vi "test Get Attribute as JSON Multiple Tables.vi"(11 "Test Case In":refnum<class "Test Config From Excel Table.lvclass">) -> (0 "error out":errorcluster, 3 "Test Case Out":refnum<class "Test Config From Excel Table.lvclass">)   [LabVIEW 2020, in "Test Config From Excel Table.lvclass"]
uses:
  Test Config From Excel Table.lvclass
  C:/Program Files/National Instruments/LabVIEW 2025/vi.lib/Astemes/LUnit/Test Case.lvclass
  Source/Config from Excel Table/Config from Excel Table.lvclass
  <vilib>/Astemes/LUnit/Test Case.lvclass/Test Case.ctl
  <vilib>/JDP Science/JSONtext/JSONtext.lvlib
  <vilib>/Astemes/LUnit/Test Case.lvclass
  <vilib>/Peter/Open Xml/Source/Open Xml.lvlib
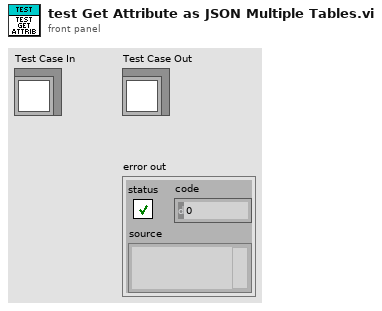
[diagram p1: front panel]
types:
  T1 = cluster{"Sheet Name":string, "Name":string, "Display Name":string, "Range or Cell Address":string}
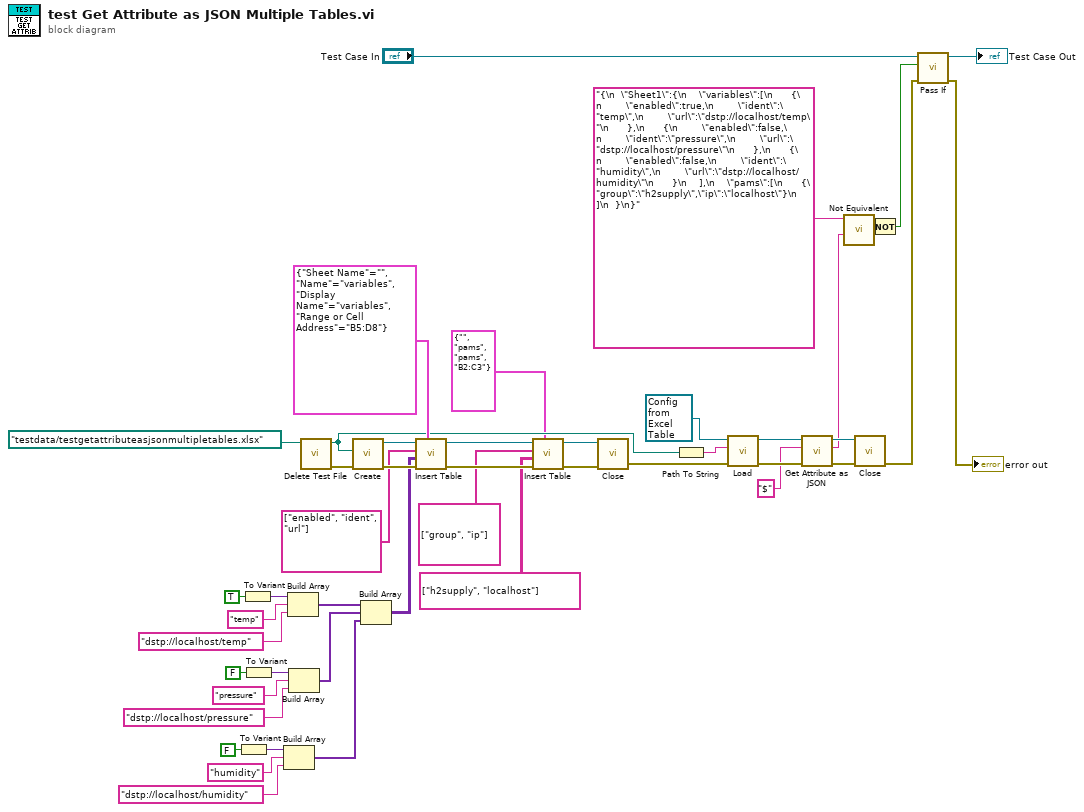
[diagram p0: block diagram]
diagram:
  n1 = To Variant(anything=FALSE) -> (Variant=w20:variant)
  n2 = To Variant(anything=TRUE) -> (Variant=w29:variant)
  n3 = To Variant(anything=FALSE) -> (Variant=w23:variant)
  n4 = Build Array(w20, "humidity", "dstp://localhost/humidity") -> (w16:variant[])
  n5 = Build Array(w29, "temp", "dstp://localhost/temp") -> (w26:variant[])
  n6 = Build Array(w23, "pressure", "dstp://localhost/pressure") -> (w17:variant[])
  n7 = call "Delete Test File.vi"("name or relative path"=path "testdata/testgetattributeasjsonmultipletables.xlsx") -> ("error out"=w34:errorcluster, "deleted path"=w9:path)  [unwired: 9 in]
  n8 = call <vilib>:"Create.vi"("error in"=w34, "Path"=w9) -> ("error out"=w33:errorcluster, "SpreadsheetDoc"=w14:refnum<k24>)  [unwired: 8 in]
  n9 = Build Array(w26, w17, w16) -> (w15:variant[][])
  n10 = call <vilib>:"Insert Table.vi"("Location"=T1 {"Sheet Name"="", "Name"="variables", "Display Name"="variables", "Range or Cell Address"="B5:D8"}, "error in"=w33, "Cell Values"=w15, "Header Names"=string[] ["enabled", "ident", "url"], "SpreadsheetDoc in"=w14) -> ("error out"=w13:errorcluster, "SpreadsheetDoc out"=w6:refnum<k24>)  [unwired: 5 in]
  n11 = call <vilib>:"Insert Table.vi"("Location"=T1 {"Sheet Name"="", "Name"="pams", "Display Name"="pams", "Range or Cell Address"="B2:C3"}, "error in"=w13, "Cell Values"=string[][] [["h2supply", "localhost"]] ("Header Names"), "Header Names"=string[] ["group", "ip"], "SpreadsheetDoc in"=w6) -> ("error out"=w7:errorcluster, "SpreadsheetDoc out"=w5:refnum<k24>)  [unwired: 5 in]
  n12 = call <vilib>:"Close.vi"("error in"=w7, "SpreadsheetDoc"=w5) -> ("error out"=w12:errorcluster)  [unwired: 9 in]
  n13 = Path To String(path=w9) -> (string=w43:string)
  n14 = call-dynamic "Load.vi"("error in"=w12, "Source"=w43, "Config from Excel Table in"=refnum<class "Config from Excel Table.lvclass"> refnum ("Config from EXCEL Table.lvclass")) -> ("error out"=w40:errorcluster, "Config from Excel Table out"=w41:refnum<class "Config from Excel Table.lvclass">)  [unwired: 7 in]
  n15 = call-dynamic "Get Attribute as JSON.vi"("error in"=w40, "Attribute"="$", "Config from Excel Table in"=w41) -> ("error out"=w38:errorcluster, "<JSON>"=w8:string, "Config from Excel Table out"=w37:refnum<class "Config from Excel Table.lvclass">)  [unwired: 6 in]
  n16 = call <vilib>:"Not Equivalent.vi"("Other JSON"=w8, "JSON"="{\n  \"Sheet1\":{\n    \"variables\":[\n      {\n        \"enabled\":true,\n        \"ident\":\"temp\",\n        \"url\":\"dstp://localhost/temp\"\n      },\n      {\n        \"enabled\":false,\n        \"ident\":\"pressure\",\n        \"url\":\"dstp://localhost/pressure\"\n      },\n      {\n        \"enabled\":false,\n        \"ident\":\"humidity\",\n        \"url\":\"dstp://localhost/humidity\"\n      }\n    ],\n    \"pams\":[\n      {\"group\":\"h2supply\",\"ip\":\"localhost\"}\n    ]\n  }\n}") -> ("Not Equivalent"=w36:bool)  [unwired: 8 in]
  n17 = call-dynamic <vilib>:"Close.vi"("error in"=w38, "Config from Excel Table in"=w37) -> ("error out"=w42:errorcluster)  [unwired: 8 in, 1 out]
  n18 = Not(x=w36) -> (.not. x?=w35:bool)
  n19 = call <vilib>:"Pass If.vi"("error in (no error)"=w42, "Pass?"=w35, "LUnit Test Case In"="Test Case In") -> ("error out"=→"error out":errorcluster, "LUnit Test Case Out"=→"Test Case Out":refnum<class "Test Config From Excel Table.lvclass">)  [unwired: 7 in]
